vi "Vecteurintersection.vi"(2 "Direction X":bool, 3 "Direction Y":bool, 4 "Actuel X":i32, 5 "vecteur Xv":sgl format="%.34f", 6 "vecteur Yv":sgl format="%.34f", 7 "Actuel Y":i32) -> (0 "Cible X":u32, 1 "Cible Y":u32)   [LabVIEW 2010]
panel:
  out "kv":sgl format="%.10f"
  out "kx":sgl format="%.10f"
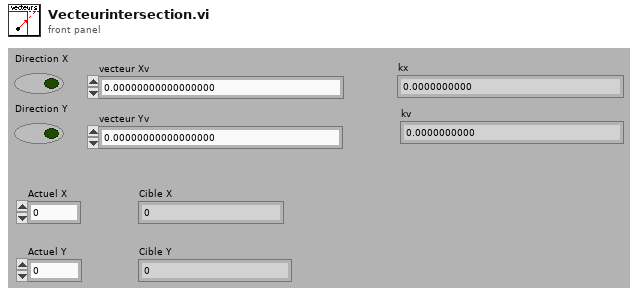
[diagram p1: front panel]
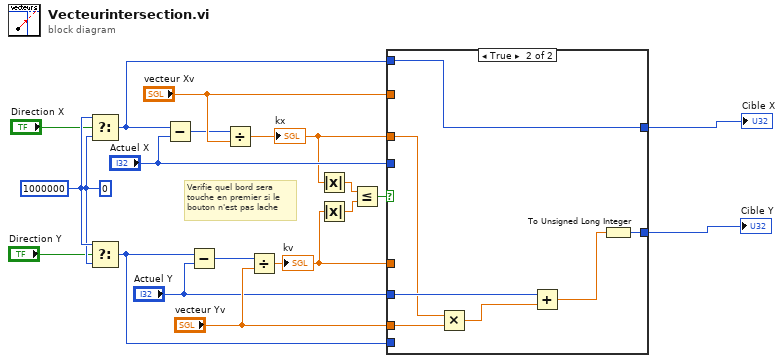
[diagram p0: block diagram]
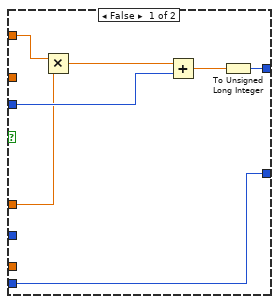
[diagram p2: hidden frame]
diagram:
  w18 = 0 ("cas vrai")
  w19 = 1000000 ("cas vrai")
  # "Verifie quel bord sera\ntouche en premier si le\nbouton n'est pas lache"
  n1 = Select(t=w19, s="Direction X", f=w18) -> (s? t:f=w9:i32)
  n2 = Select(t=w19, s="Direction Y", f=w18) -> (s? t:f=w10:i32)
  n3 = Subtract(x=w9, y="Actuel X") -> (x-y=w1:i32)
  n4 = Subtract(x=w10, y="Actuel Y") -> (x-y=w2:i32)
  n5 = Divide(x=w1, y="vecteur Xv") -> (x/y=w7:sgl)
  "kx" <- w7
  n6 = Divide(x=w2, y="vecteur Yv") -> (x/y=w5:sgl)
  "kv" <- w5
  n7 = Absolute Value(x=w7) -> (abs(x)=w8:sgl)
  n8 = Absolute Value(x=w5) -> (abs(x)=w6:sgl)
  n9 = Less Or Equal?(x=w8, y=w6) -> (x <= y?=w17:bool)
  n10 = case shown="True" w17 {
    tunnel: "vecteur Yv" -> [_ w32]
    tunnel: "Actuel Y" -> [_ w31]
    tunnel: w5 -> [w21 _]
    tunnel: "vecteur Xv" -> [w25 _]
    tunnel: "Actuel X" -> [w23 _]
    tunnel: w7 -> [_ w28]
    tunnel: w10 -> [w26 _]
    tunnel: w9 -> [_ w33]
    tunnel: [w20 w33] -> w4
    tunnel: [w26 w27] -> w3
    frame False {
      n11 = Multiply(x=w25, y=w21) -> (x*y=w22:sgl)
      n12 = Add(x=w22, y=w23) -> (x+y=w24:sgl)
      n13 = To Unsigned Long Integer(number=w24) -> (unsigned 32bit integer=w20:u32)
    }
    frame True {
      n14 = Multiply(x=w28, y=w32) -> (x*y=w30:sgl)
      n15 = Add(x=w31, y=w30) -> (x+y=w29:sgl)
      n16 = To Unsigned Long Integer(number=w29) -> (unsigned 32bit integer=w27:u32)
    }
  }
  "Cible X" <- w4
  "Cible Y" <- w3
